vi "convert-to-binary-block.vi"(1 "Array to Binary Block Format":dbl[](array[numeric])) -> (0 "Binary Block":string)   [LabVIEW 2013]
doc: "Feed in an array of values between -1 and 1\n- Generates a binary block\n- Write to keysight with :DATA:DAC VOLATILE command\n- Write to persistent memeory (after writting first to VOLATILE) with :DATA:COPY <<NAME>>, VOLATILE\n- Delete with :DATA:DEL <<NAME>>"
panel:
  out "Binary representation":u16[](array[numeric])
  out "Hex representation":string
  out "String representation":string
  out "Binary Representation":bool[](array[boolean])
  out "Length of binary block (in bytes)":i32
  # ":DATA:DAC VOLTATILE\n:DATA:COPY RANDOM-NAME, VOLATILE"
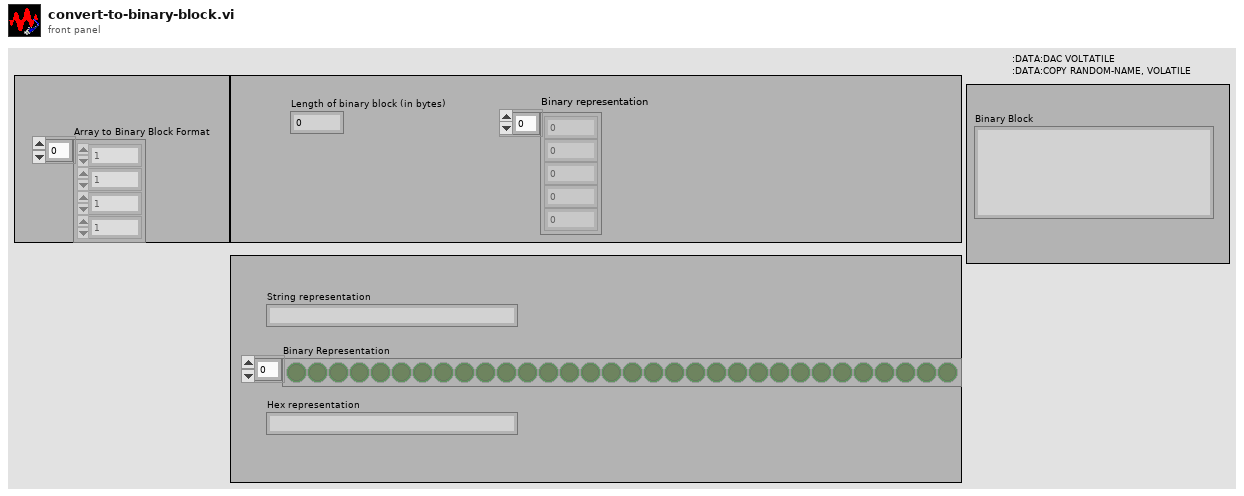
[diagram p1: front panel]
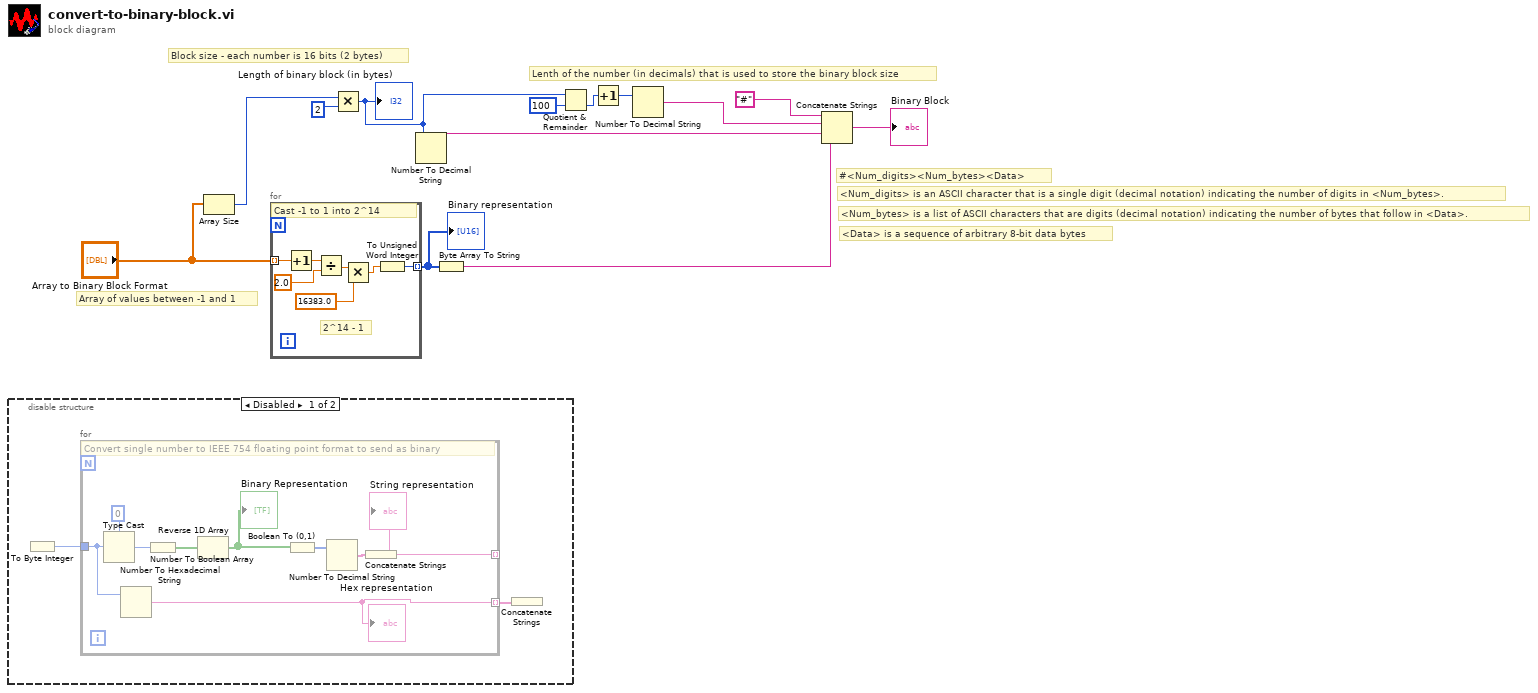
[diagram p0: block diagram]
diagram:
  # "Array of values between -1 and 1"
  # "<Data> is a sequence of arbitrary 8-bit data bytes"
  # "<Num_bytes> is a list of ASCII characters that are digits (decimal notation) indicating the number of bytes that follow in <Data>."
  # "<Num_digits> is an ASCII character that is a single digit (decimal notation) indicating the number of digits in <Num_bytes>."
  # "#<Num_digits><Num_bytes><Data>"
  # "Block size - each number is 16 bits (2 bytes)"
  # "Lenth of the number (in decimals) that is used to store the binary block size"
  n1 = disable-structure shown="Disabled" {
    frame Disabled {
      n2 = To Byte Integer() -> (8bit integer=w14:i8)  [unwired: 1 in]
      n3 = for {
        tunnel: w14 -> [w17]
        tunnel: [w18] -> _ mode=indexing
        tunnel: [w16] -> w15 mode=indexing
        # "Convert single number to IEEE 754 floating point format to send as binary"
        n4 = Type Cast(type=0 ("Numeric"), x=w17) -> (*(type *) &x=w20:i32)
        n5 = Number To Hexadecimal String(2:w17) -> (0:w16:string)  [unwired: 1 in]
        "Hex representation" <- w16
        n6 = Number To Boolean Array(number=w20) -> (Boolean array=w21:bool[])
        n7 = Reverse 1D Array(array=w21) -> (reversed array=w24:bool[])
        "Binary Representation" <- w24
        n8 = Boolean To (0,1)(Boolean=w24) -> (0, 1=w22:i16[])
        n9 = Number To Decimal String(number=w22) -> (decimal integer string=w23:string[])  [unwired: 1 in]
        n10 = Concatenate Strings(w23) -> (w18:string)
        "String representation" <- w18
      }
      n11 = Concatenate Strings(w15) -> ()  [unwired: 1 out]
    }
    frame Enabled {
    }
  }
  n12 = Array Size(array="Array to Binary Block Format") -> (size(s)=w10:i32)
  n13 = for {
    tunnel: "Array to Binary Block Format" -> [w30] mode=indexing
    tunnel: [w27] -> w1 mode=indexing
    # "2^14 - 1"
    # "Cast -1 to 1 into 2^14"
    n14 = Increment(x=w30) -> (x+1=w26:dbl)
    n15 = Divide(x=w26, y=2.0) -> ()  [unwired: 1 out]
    n16 = Multiply(x=w26, y=16383.0) -> (x*y=w28:dbl)
    n17 = To Unsigned Word Integer(number=w28) -> (unsigned 16bit integer=w27:u16)
  }
  "Binary representation" <- w1
  n18 = Multiply(x=w10, y=2) -> (x*y=w8:i32)
  "Length of binary block (in bytes)" <- w8
  n19 = Number To Decimal String(number=w8) -> (decimal integer string=w12:string)  [unwired: 1 in]
  n20 = Byte Array To String(unsigned byte array=w1) -> (string=w3:string)
  n21 = Quotient & Remainder(x=w8, y=100) -> (floor(x/y)=w5:i32)  [unwired: 1 out]
  n22 = Increment(x=w5) -> (x+1=w4:i32)
  n23 = Number To Decimal String(number=w4) -> (decimal integer string=w6:string)  [unwired: 1 in]
  n24 = Concatenate Strings("#" ("string"), w6, w12, w3) -> (→"Binary Block":string)
